vi "Add Waveform to List.vi"(7 "Waveform List Ctl Ref":refnum<vi>, 8 "error in (no error)":errorcluster, 10 "Waveform to Add":waveform(dbl), 11 "Canvas Wfm Array In":waveform(dbl)[](array[waveform])) -> (0 "error out":errorcluster, 3 "Canvas Wfm Array Out":waveform(dbl)[](array[waveform]))   [LabVIEW 2025, in "TDMS Waveform Creator UI.lvlib"]
uses:
  TDMS Waveform Creator UI.lvlib
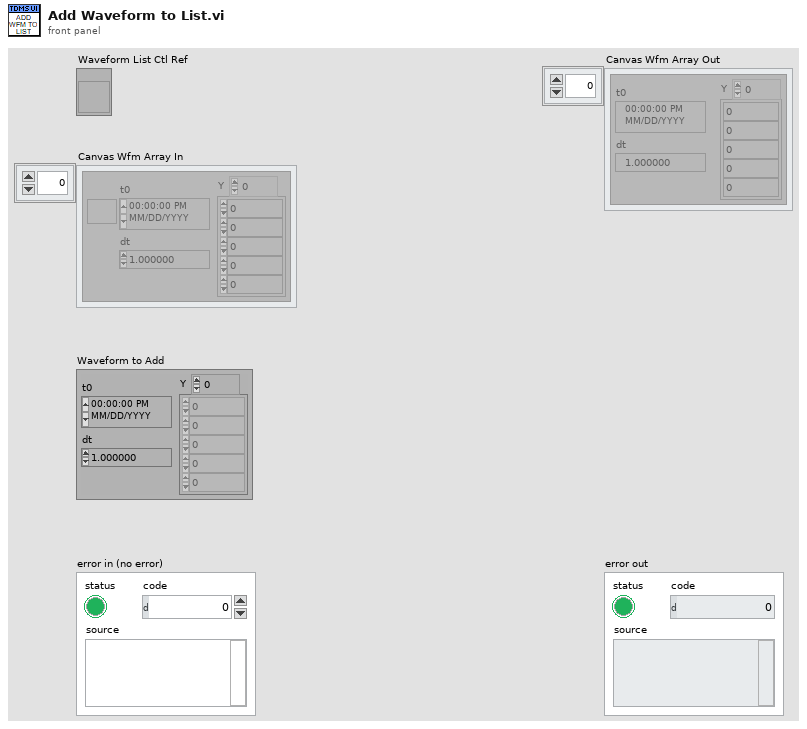
[diagram p1: front panel]
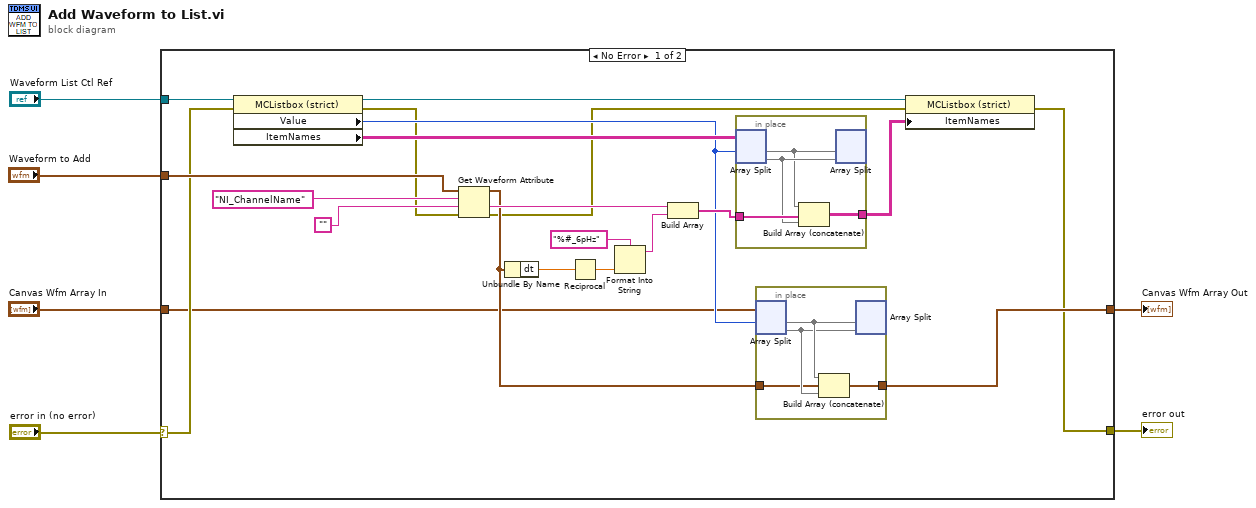
[diagram p0: block diagram]
diagram:
  n1 = case shown="No Error" "error in (no error)" {
    selector: "error in (no error)" -> [w12 w37]
    tunnel: "Waveform to Add" -> [w27 _]
    tunnel: "Waveform List Ctl Ref" -> [w26 _]
    tunnel: "Canvas Wfm Array In" -> [w9 w36]
    tunnel: [w8 w36] -> w2
    tunnel: [w7 w37] -> w1
    frame No Error {
      n2 = property class="MCListbox (strict)"(reference=w26, error in=w12) -> (reference out=w16:refnum<vi>, error out=w11:errorcluster, "Value"=w14:i32, "ItemNames"=w25:string[][])
      n3 = Get Waveform Attribute(4:w11, 5:"", 6:"NI_ChannelName" ("name"), 7:w27) -> (0:w10:errorcluster, 1:w19:string, 3:w13:waveform(dbl))  [unwired: 1 out]
      n4 = Unbundle By Name(w13) -> ("dt"=w22:dbl)
      n5 = Reciprocal(x=w22) -> (1/x=w21:dbl)
      n6 = Format Into String(format string="%#_6pHz", w21) -> (resulting string=w18:string)  [unwired: 2 in, 1 out]
      n7 = Build Array(w19, w18) -> (w17:string[])
      n8 = in-place {
        in-place-border: w17 -> [w31]
        in-place-border: [w30] -> w15
        n9 = in-place-split #1(w25, w14) -> (w28:string[][], w29:string[][])
        n10 = Build Array (concatenate)(w28, w31, w29) -> (w30:string[][])
        n11 = in-place-split #1(w28, w29) -> ()  [unwired: 2 out]
      }
      n12 = in-place {
        in-place-border: [w35] -> w8
        in-place-border: w13 -> [w32]
        n13 = in-place-split #2(w9, w14) -> (w34:waveform(dbl)[], w33:waveform(dbl)[])
        n14 = Build Array (concatenate)(w34, w32, w33) -> (w35:waveform(dbl)[])
        n15 = in-place-split #2(w34, w33) -> ()  [unwired: 2 out]
      }
      n16 = property class="MCListbox (strict)"(reference=w16, error in=w10, "ItemNames"=w15) -> (error out=w7:errorcluster)  [unwired: 1 out]
    }
    frame Error {
    }
  }
  "error out" <- w1
  "Canvas Wfm Array Out" <- w2
